vi "graficos.vi"() -> ()   [LabVIEW 2019]
panel:
  in  "Boolean":bool
  out "Waveform Graph":dbl[](graph)
  out "Waveform Chart":dbl(graph)
  in  "stop":bool
  in  "Slide":dbl(slide) scale=0.0..50.0
  out "Thermometer":dbl(slide) scale=0.0..50.0
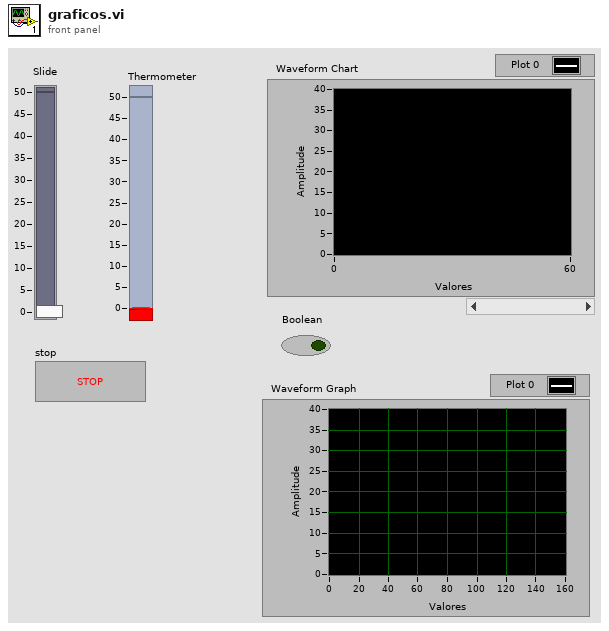
[diagram p1: front panel]
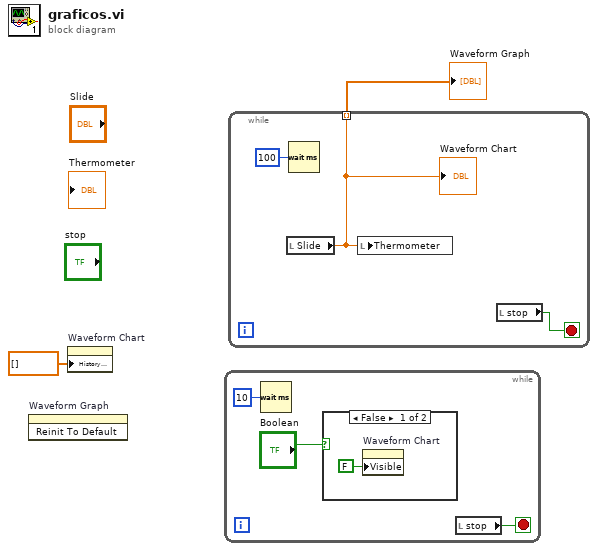
[diagram p0: block diagram]
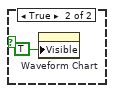
[diagram p2: hidden frame]
diagram:
  n1 = invoke on="Waveform Graph" class="WFGraph (strict)" method="Reinit To Default"() -> ()  [unwired: 3 in, 3 out]
  n2 = property on="Waveform Chart" class="WFChart (strict)"("History Data"=dbl[] []) -> ()  [unwired: 2 in, 2 out]
  n3 = while {
    stop <- w4 stop-if-true
    n4 = Wait (ms)(milliseconds to wait=u32 10) -> ()  [unwired: 1 out]
    n5 = case shown="False" "Boolean" {
      frame False {
        n6 = property on="Waveform Chart" class="WFChart (strict)"("Visible"=FALSE) -> ()  [unwired: 2 in, 2 out]
      }
      frame True {
        n7 = property on="Waveform Chart" class="WFChart (strict)"("Visible"=TRUE) -> ()  [unwired: 2 in, 2 out]
      }
    }
    n8 = local read "stop"() -> (w4:bool)
  }
  n9 = while {
    tunnel: [w8] -> w2 mode=indexing
    stop <- w9 stop-if-true
    n10 = local read "Slide"() -> (w8:dbl)
    "Waveform Chart" <- w8
    n11 = Wait (ms)(milliseconds to wait=u32 100) -> ()  [unwired: 1 out]
    n12 = local write "Thermometer"(w8) -> ()
    n13 = local read "stop"() -> (w9:bool)
  }
  "Waveform Graph" <- w2
